vi "DllFxpDivTemp.vi"(6 "ready for output":bool, 9 "input valid":bool, 10 "y":fxp<+/-,64,32>, 11 "x":fxp<+/-,64,32>) -> (1 "output valid":bool, 2 "overflow?":bool, 3 "x/y":fxp<+,1,1>, 4 "ready for input":bool)   [LabVIEW 2017]
uses:
  <vilib>/rvi/FXPMathLib/FxpDiv/subVIs/nifxpmath_Div_SimConfig.ctl
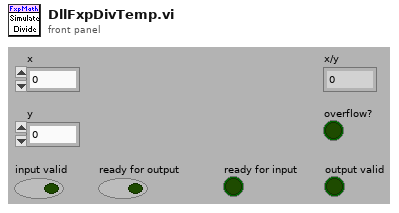
[diagram p1: front panel]
types:
  T1 = typedef "nifxpmath_Div_SimConfig.ctl" = cluster{"kXSigned":bool, "kXWl":u32, "kXIwl":i32, "kYSigned":bool, "kYWl":u32, "kYIwl":i32, "kZSigned":bool, "kZWl":u32, "kZIwl":i32, "Saturate":bool, "SupportSCTL?":bool, "Limit of Iterations":u16, "Strict Limit?":bool, "InputRegister":bool, "OutputRegister":bool}
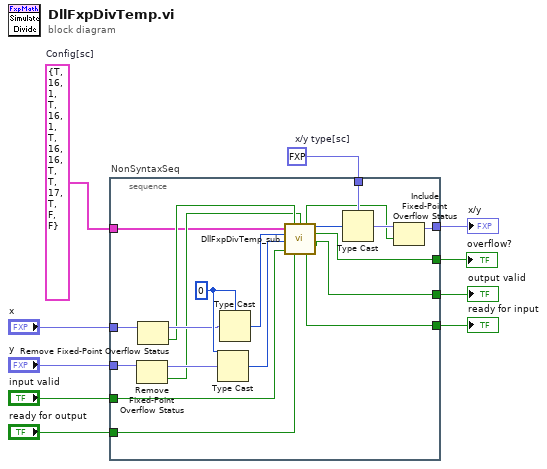
[diagram p0: block diagram]
diagram:
  w1 = T1 {"kXSigned"=TRUE, "kXWl"=16, "kXIwl"=1, "kYSigned"=TRUE, "kYWl"=16, "kYIwl"=1, "kZSigned"=TRUE, "kZWl"=16, "kZIwl"=16, "Saturate"=TRUE, "SupportSCTL?"=TRUE, "Limit of Iterations"=17, "Strict Limit?"=TRUE, "InputRegister"=FALSE, "OutputRegister"=FALSE}  # Config[sc]
  w8 = fxp<+,1,1> 0.0  # x/y type[sc]
  n1 = stacked-sequence "NonSyntaxSeq" {
    tunnel: "x" -> [w20]
    tunnel: "y" -> [w17]
    tunnel: w8 -> [w30]
    tunnel: [w12] -> w7
    tunnel: "input valid" -> [w26]
    tunnel: [w24] -> w5
    tunnel: [w22] -> w4
    tunnel: [w21] -> w3
    tunnel: "ready for output" -> [w23]
    tunnel: w1 -> [w11]
    frame #0 {
      w29 = u64 0
      n2 = Remove Fixed-Point Overflow Status(3:w17) -> (0:w15:bool, 1:w16:fxp<+/-,64,32>)
      n3 = Remove Fixed-Point Overflow Status(3:w20) -> (0:w18:bool, 1:w19:fxp<+/-,64,32>)
      n4 = Type Cast(type=w29, x=w16) -> (*(type *) &x=w27:u64)
      n5 = Type Cast(type=w29, x=w19) -> (*(type *) &x=w28:u64)
      n6 = call <vilib>:"DllFxpDivTemp_sub.vi"("Config[sc]"=w11, "x ovfl status"=w18, "y ovfl status"=w15, "x"=w28, "y"=w27, "input valid"=w26, "ready for output"=w23) -> ("x/y ovfl status"=w13:bool, "x/y"=w25:u64, "operational overflow"=w24:bool, "output valid"=w21:bool, "ready for input"=w22:bool)  [unwired: 4 out]
      n7 = Type Cast(type=w30, x=w25) -> (*(type *) &x=w14:fxp<+,1,1>)
      n8 = Include Fixed-Point Overflow Status(2:w13, 3:w14) -> (1:w12:fxp<+,1,1>)
    }
  }
  "overflow?" <- w5
  "x/y" <- w7
  "output valid" <- w3
  "ready for input" <- w4
